vi "Image Transfer FPGA to RT (SubVI).vi"(8 "error in (no error)":errorcluster, 9 "Refnum in":T1, 10 "Image Size Out":T2, 11 "Custom FPGA Reference In":refnum<k20>) -> (0 "error out":errorcluster, 1 "Elements Remaining":u32, 2 "Image Out":T1, 3 "Custom FPGA Reference Out":refnum<k20>)   [LabVIEW 2017]
uses:
  Controls/Image Size.ctl
  <vilib>/vision/Image Controls.llb/IMAQ Image.ctl
  <vilib>/Utility/error.llb/Error Cluster From Error Code.vi
  <vilib>/rvi/errors/niLvFpgaAdjustHostInterfaceError.vi
  <vilib>/rvi/interface/nirviMethod/nirviMethod.xnode
  <vilib>/vision/NI_Vision_Development_Module.lvlib
  <vilib>/FPGAPlugInAG/Dynamic/niLvFpga_ReadFifo_Dynamic.vi
  <vilib>/rvi/errors/niLvFpgaMergeErrorWithErrorCode.vi
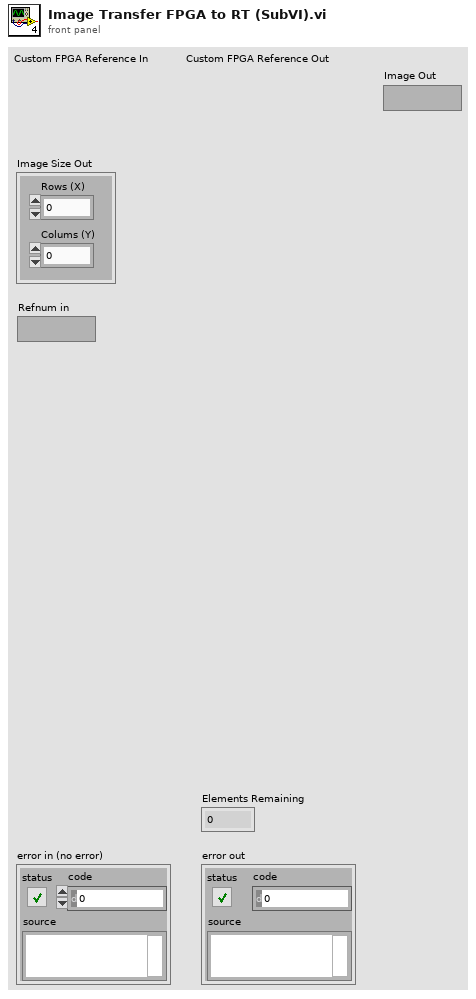
[diagram p1: front panel]
types:
  T1 = typedef "IMAQ Image.ctl" = refnum<image>
  T2 = typedef "Image Size.ctl" = cluster{"Rows (X)":u16, "Colums (Y)":u16}
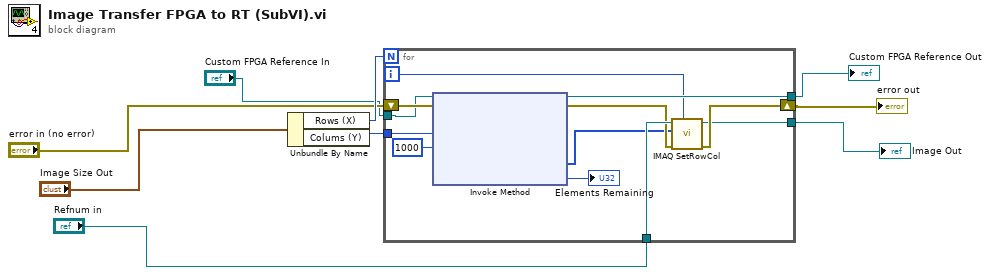
[diagram p0: block diagram]
diagram:
  n1 = Unbundle By Name("Image Size Out") -> ("Rows (X)"=w9:u16, "Colums (Y)"=w7:u16)
  n2 = for {
    N: w9 -> [_]
    shift-right: [w13] -> w5
    shift-left: "error in (no error)" -> [w18]
    tunnel: [w21] -> w1
    tunnel: "Refnum in" -> [w17]
    tunnel: w7 -> [w12]
    tunnel: [w11] -> w3
    tunnel: "Custom FPGA Reference In" -> [w10]
    i -> [w14]
    n3 = xnode "Invoke Method"("FPGA VI Reference In"=w10, "error in"=w18, "Number of Elements"=w12, "Timeout (ms)"=1000) -> ("FPGA VI Reference Out"=w21:refnum<k20>, "error out"=w16:errorcluster, "Data"=w15:u8[], "Elements Remaining"=→"Elements Remaining":u32)
    n4 = call "IMAQ SetRowCol"("Number"=w14, "error in (no error)"=w16, "Pixels (U8)"=w15, "Image"=w17) -> ("error out"=w13:errorcluster, "Image Out"=w11:T1)  [unwired: 6 in]
  }
  "error out" <- w5
  "Image Out" <- w3
  "Custom FPGA Reference Out" <- w1
